vi "OnDataDrag3.vi"(0 "XRef":T21, 1 "Point":T19, 2 "String":T13, 3 "Path":T18, 4 "ProjectItemRefs":T16, 5 "GObjRefs":T14, 6 "State In":T1) -> (14 "Reply":T12, 15 "Fatal Error Out":T11, 16 "State Out":T1)   [LabVIEW 2020, in "Parallel Diagram Block.xnode"]
uses:
  Parallel Diagram Block.xnode
  <vilib>/XNodeSupport/XNodeString.ctl
  <vilib>/XNodeSupport/NI_XNodeSupport.lvlib
  <vilib>/XNodeSupport/XNodeStringArray.ctl
  Parallel Block/Type Descriptor/Type Descriptor.lvclass
  Parallel Block/Block/Block.lvclass
  <vilib>/XNodeSupport/XNodeXNodeRef.ctl
  <vilib>/XNodeSupport/XNodeInt.ctl
  <vilib>/XNodeSupport/XNodePoint.ctl
  <vilib>/XNodeSupport/XNodePath.ctl
  <vilib>/XNodeSupport/XNodeProjItemRef.ctl
  <vilib>/XNodeSupport/XNodeProjItemRefArray.ctl
  <vilib>/XNodeSupport/XNodeGObjRef.ctl
  <vilib>/XNodeSupport/XNodeGObjRefArray.ctl
  <vilib>/XNodeSupport/XNodeErrorCluster.ctl
  State.ctl
  Parallel Block/Value Type.ctl
  Parallel Block/Parallel Block.lvlib
  Parallel Block/Type Descriptor.ctl
  <vilib>/picture/picture.llb/imagedata.ctl
  Parallel Block/Direction.ctl
  Parallel Block/Terminal Mode.ctl
  Parallel Block/Terminal Type.ctl
  Parallel Block/Type Mode.ctl
  Parallel Block/Value Mode.ctl
  Parallel Block/Manager Node.ctl
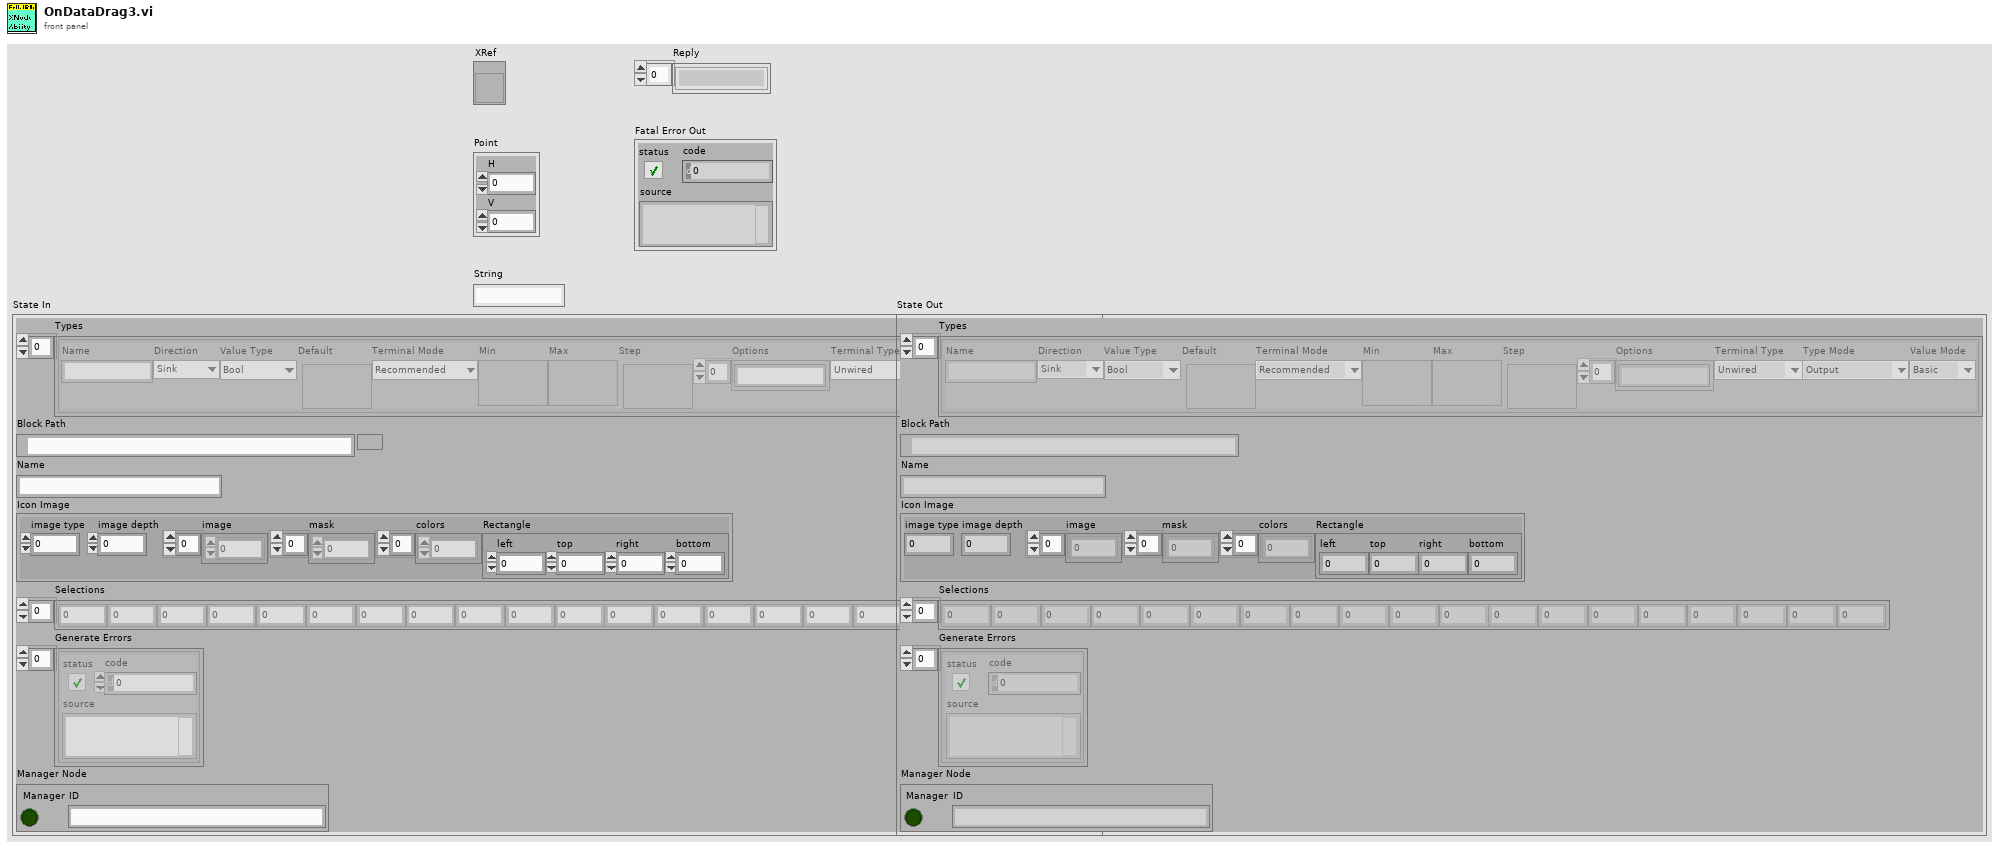
[diagram p1: front panel]
types:
  T1 = typedef "Parallel Diagram Block.xnode/State.ctl" = cluster{"Types":T2[], "Block Path":path, "Name":string, "Icon Image":T9, "Selections":i32[], "Generate Errors":errorcluster[], "Manager Node":T10}
  T2 = typedef "Parallel Block.lvlib/Type Descriptor.ctl" = cluster{"Name":string, "Direction":T3, "Value Type":T4, "Default":variant, "Terminal Mode":T5, "Min":variant, "Max":variant, "Step":variant, "Options":string[], "Terminal Type":T6, "Type Mode":T7, "Value Mode":T8}
  T3 = typedef "Parallel Block.lvlib/Direction.ctl" = enum16{"Sink", "Source"}
  T4 = typedef "Parallel Block.lvlib/Value Type.ctl" = enum16{"Unknown", "Bool", "U8", "U16", "U32", "U64", "I8", "I16", "I32", "I64", "SGL", "DBL", "CSG", "CDB", "CDBWfm", "String", "DBLWfm"}
  T5 = typedef "Parallel Block.lvlib/Terminal Mode.ctl" = enum16{"Recommended", "Required", "None"}
  T6 = typedef "Parallel Block.lvlib/Terminal Type.ctl" = enum16{"Unwired", "BadType", "Connection", "Value", "Control Ref", "BadRefType"}
  T7 = typedef "Parallel Block.lvlib/Type Mode.ctl" = enum16{"Output", "Single - Strict", "Single - Coerced", "Stream"}
  T8 = typedef "Parallel Block.lvlib/Value Mode.ctl" = enum16{"Basic", "Range", "Select"}
  T9 = typedef "imagedata.ctl" = cluster{"image type":i32, "image depth":i32, "image":u8[], "mask":u8[], "colors":u32[], "Rectangle":cluster{"left":i16, "top":i16, "right":i16, "bottom":i16}}
  T10 = typedef "Parallel Block.lvlib/Manager Node.ctl" = cluster{"Manager":bool, "ID":string}
  T11 = typedef "NI_XNodeSupport.lvlib/XNodeErrorCluster.ctl" = errorcluster
  T12 = typedef "NI_XNodeSupport.lvlib/XNodeStringArray.ctl" = T13[]
  T13 = typedef "NI_XNodeSupport.lvlib/XNodeString.ctl" = string
  T14 = typedef "NI_XNodeSupport.lvlib/XNodeGObjRefArray.ctl" = T15[]
  T15 = typedef "NI_XNodeSupport.lvlib/XNodeGObjRef.ctl" = refnum<vi>
  T16 = typedef "NI_XNodeSupport.lvlib/XNodeProjItemRefArray.ctl" = T17[]
  T17 = typedef "NI_XNodeSupport.lvlib/XNodeProjItemRef.ctl" = refnum<vi>
  T18 = typedef "NI_XNodeSupport.lvlib/XNodePath.ctl" = path
  T19 = typedef "NI_XNodeSupport.lvlib/XNodePoint.ctl" = cluster{"H":T20, "V":T20}
  T20 = typedef "NI_XNodeSupport.lvlib/XNodeInt.ctl" = i32
  T21 = typedef "NI_XNodeSupport.lvlib/XNodeXNodeRef.ctl" = refnum<vi>
  T22 = enum32{"invalid scope", "public", "private", "protected", "community"}
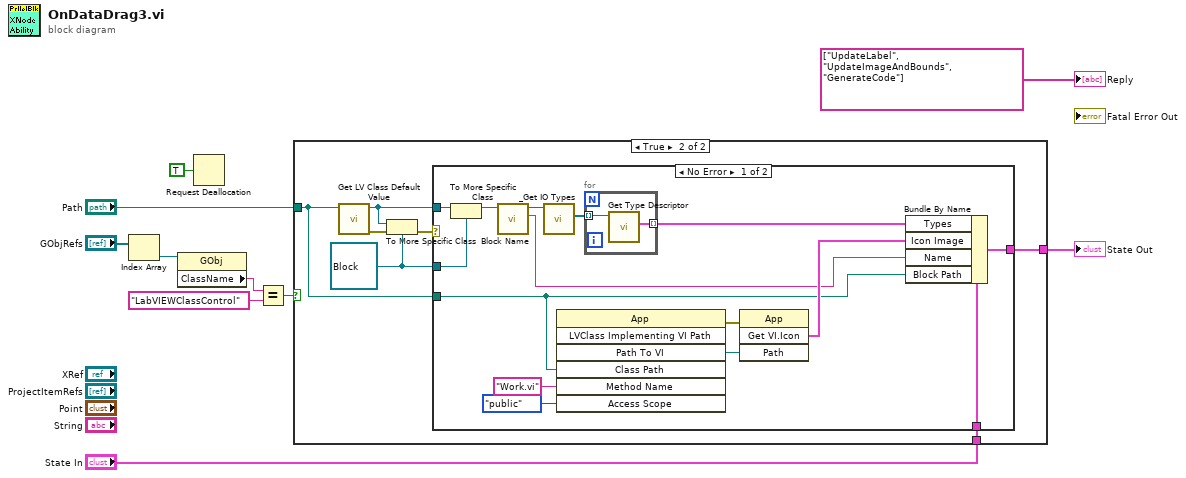
[diagram p0: block diagram]
diagram:
  n1 = Index Array(array="GObjRefs") -> (element=w7:T15)  [unwired: 1 in]
  n2 = property class="GObj"(reference=w7) -> ("ClassName"=w6:string)  [unwired: 1 in, 2 out]
  n3 = Request Deallocation(TRUE ("flag")) -> ()
  n4 = Equal?(x=w6, y="LabVIEWClassControl") -> (x = y?=w4:bool)
  n5 = case shown="True" w4 {
    tunnel: "Path" -> [_ w14]
    tunnel: "State In" -> [w11 w16]
    tunnel: [w11 w15] -> w1
    frame False {
    }
    frame True {
      w12 = refnum<class "Block.lvclass"> refnum ("Parallel Block.lvlib:Block.lvclass")
      n6 = call <vilib>:"Get LV Class Default Value.vi"("class path"=w14) -> ("error out"=w18:errorcluster, "object"=w13:refnum<class>)  [unwired: 9 in]
      n7 = To More Specific Class(target class=w12, reference=w13, error in=w18) -> (error out=w17:errorcluster)  [unwired: 1 out]
      n8 = case shown="No Error" w17 {
        tunnel: w13 -> [w22 _]
        tunnel: w16 -> [w33 w36]
        tunnel: [w32 w36] -> w15
        tunnel: w14 -> [w25 _]
        tunnel: w12 -> [w20 _]
        frame No Error {
          n9 = To More Specific Class(target class=w20, reference=w22) -> (specific class reference=w21:refnum<class "Block.lvclass">)  [unwired: 1 in, 1 out]
          n10 = call-dynamic "Block Name.vi"("Block in"=w21) -> ("Name"=w23:string, "Block out"=w24:refnum<class "Block.lvclass">)  [unwired: 8 in, 1 out]
          n11 = call "_Get IO Types.vi"("Block in"=w24) -> ("Types"=w31:refnum<class "Type Descriptor.lvclass">[])  [unwired: 8 in, 2 out]
          n12 = invoke class="App" method="LVClass Implementing VI Path"("Class Path"=w25, "Method Name"="Work.vi", "Access Scope"=T22."public") -> (error out=w27:errorcluster, "Path To VI"=w28:path)  [unwired: 4 in, 5 out]
          n13 = for {
            tunnel: w31 -> [w34] mode=indexing
            tunnel: [w35] -> w19 mode=indexing
            n14 = call "Get Type Descriptor.vi"("Type Descriptor in"=w34) -> ("Type Descriptor"=w35:T2)  [unwired: 8 in, 2 out]
          }
          n15 = invoke class="App" method="Get VI.Icon"(error in=w27, "Path"=w28) -> ("Get VI.Icon"=w26:T9)  [unwired: 2 in, 3 out]
          n16 = Bundle By Name(cluster=w33, "Types"=w19, "Icon Image"=w26, "Name"=w23, "Block Path"=w25) -> (w32:T1)
        }
        frame Error {
        }
      }
    }
  }
  "State Out" <- w1
  "Reply" <- T12 ["UpdateLabel", "UpdateImageAndBounds", "GenerateCode"] ("Reply")
